vi "ncs_v2.vi"() -> ()   [LabVIEW 2016]
uses:
  <instrlib>/niUSRP/niUSRP Timestamp.ctl
  <vilib>/Analysis/coordinate.llb/Wrap Angle (array).vi
  <instrlib>/niUSRP/niUSRP Configure Time Start Trigger.vi
  <vilib>/Analysis/3filter.llb/Butterworth Filter (DBL).vi
  <instrlib>/niUSRP/niUSRP Fetch Rx Data (2D CDB).vi
  <vilib>/measure/maspectr.llb/FFT Power Spectrum for 1 Chan (CDB).vi
  <instrlib>/niUSRP/niUSRP Write Tx Data (2D CDB).vi
  <vilib>/measure/NI_MABase.lvlib
  <vilib>/measure/NI_MAPro.lvlib
  <vilib>/Analysis/NI_AALBase.lvlib
  <vilib>/Analysis/NI_AALPro.lvlib
  <vilib>/Analysis/NI_AAL_Angle.lvlib
panel:
  in  "File Name":string="Test"
  in  "order1":i32=5
  in  "Order":dbl=20.0 format="%#_13g"
  in  "Path":path=path "D:/Research/SummerFall17Spring18/CnC/NCS/MotionDetectionSleep/MyExperiment/Labview"
  in  "Low-Pass Freq":dbl=200.0 format="%#_13g"
  out "NCS magnitude filtered":dbl[](graph)
  in  "High-Cutoff":dbl=8.0 format="%#_13g"
  in  "Initialize Array-based filter":bool
  in  "Low-Cutoff":dbl=0.5 format="%#_13g"
  in  "Sampling Rate":i32=500
  out "Gain":dbl=-15.0
  out "Bandwidth":dbl=56000000.0
  out "Coerced Carrier Frequency":dbl=2000000000.0 format="%#.17g"
  out "Coerced Tx IQ rate":dbl=1000000.0
  out "Coerced Rx IQ rate":dbl=1000000.0
  out "error IO":errorcluster={"status"=FALSE, "code"=-1074118647, "source"=""}
  in  "Rx Number of Samples":i32=20000
  in  "Tab Control 2":enum32{"NI-294x/295x", "NI-2900/2901"}(tab)=enum."NI-2900/2901"
  in  "channel 0 carrier\n frequency [Hz]":dbl=2000000000.0 format="%#_6p"
  in  "Rx carrier frequency [Hz]":dbl=2000000000.0 format="%#_6p"
  in  "Tx carrier frequency [Hz]":dbl=1000000000.0 format="%#_6p"
  in  "Start Trigger Time":T1={"whole seconds"=1, "fractional seconds"=0.0}
  out "Tx Active Antenna":string="TX1"
  in  "Tab Control":T2(tab)
  out "NCS tag Amp":dbl[](graph)=[0.011967714738528729, 0.012021355192189592, 0.012015275039596582, 0.011969166030167903, 0.011958890166168242, 0.012007893820858737, 0.012022893722444085, 0.011978222225113794, 0.011969989939463181, 0.012003099640895068]
  out "NCS tag Phase":dbl[](graph)=[0.011967714738528729, 0.012021355192189592, 0.012015275039596582, 0.011969166030167903, 0.011958890166168242, 0.012007893820858737, 0.012022893722444085, 0.011978222225113794, 0.011969989939463181, 0.012003099640895068]
  out "IQ":dbl[][](graph)
  out "Tag Amp":dbl[](graph)
  out "Tag Phase":dbl[](graph)
  out "Baseband Power Spectrum":cluster{"f0":dbl, "df":dbl, "magnitude":dbl[]}[](graph)
  in  "Stop":bool
  in  "Channel 0\nTone Amplitude":dbl=0.707 step=0.05 format="%#.6g"
  in  "Channel 0 \nTone Frequency":dbl=5000.0 format="%#_6p"
  out "Tx Waveform Graph":waveform(dbl)[](graph)
  in  "Waveform Size":dbl=2000.0
  in  "Rx Active Antenna":string="RX2"
  in  "Device Name":refnum<k15>="MyB200"
  in  "Tx Gain":dbl=28.0 format="%#_6f"
  in  "Tx IQ Rate":dbl=1000000.0 format="%#_6p"
  in  "Rx Gain":dbl=32.0 format="%#_6f"
  in  "Rx IQ Rate":dbl=1000000.0 format="%#_6p"
  # "Rx Settings"
  # "Tx Settings"
  # "Note that on the NI-2900 and NI-2901, both Rx channels share an LO and both Tx channels share an LO. However, on the NI-294x/295x devices, Rx and Tx of channel 0 share an LO and Rx and Tx of channel 1 share an LO."
  # "This Tx graph should always have end and start tied up since this is being sent in a loop continuously. Otherwise phase jumps will be noticed."
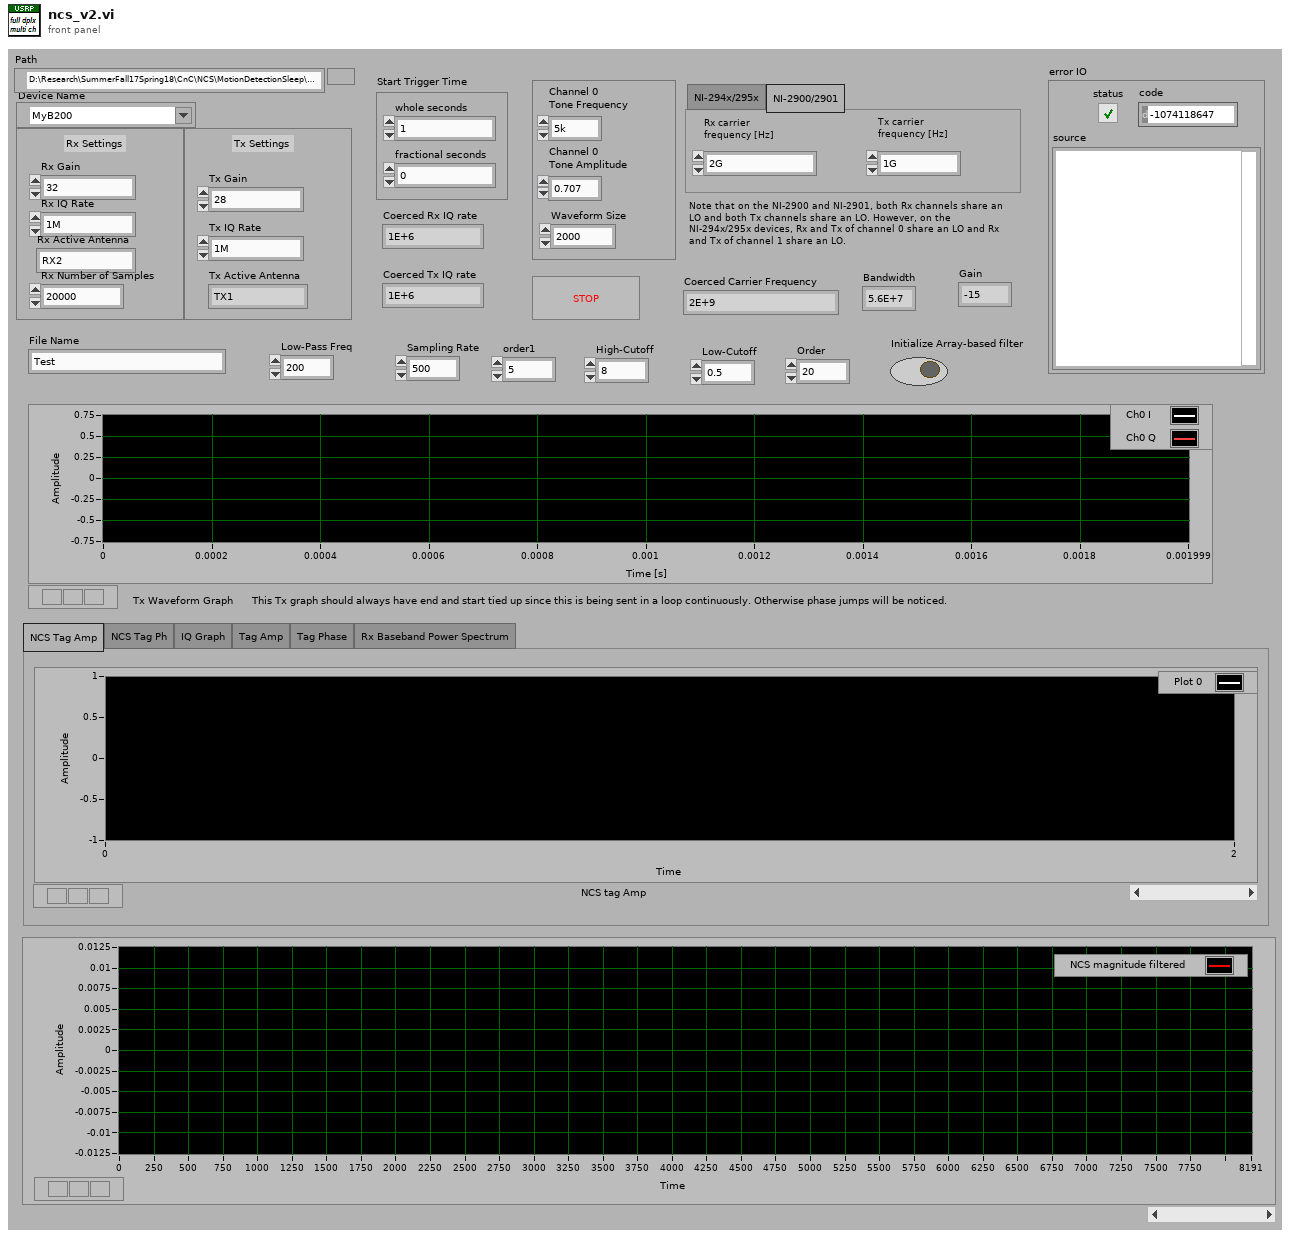
[diagram p1: front panel]
types:
  T1 = typedef "niUSRP Timestamp.ctl" = cluster{"whole seconds":u64, "fractional seconds":dbl}
  T2 = enum32{"NCS Tag Amp", "NCS Tag Ph", "IQ Graph", "Tag Amp", "Tag Phase", "Rx Baseband Power Spectrum"}
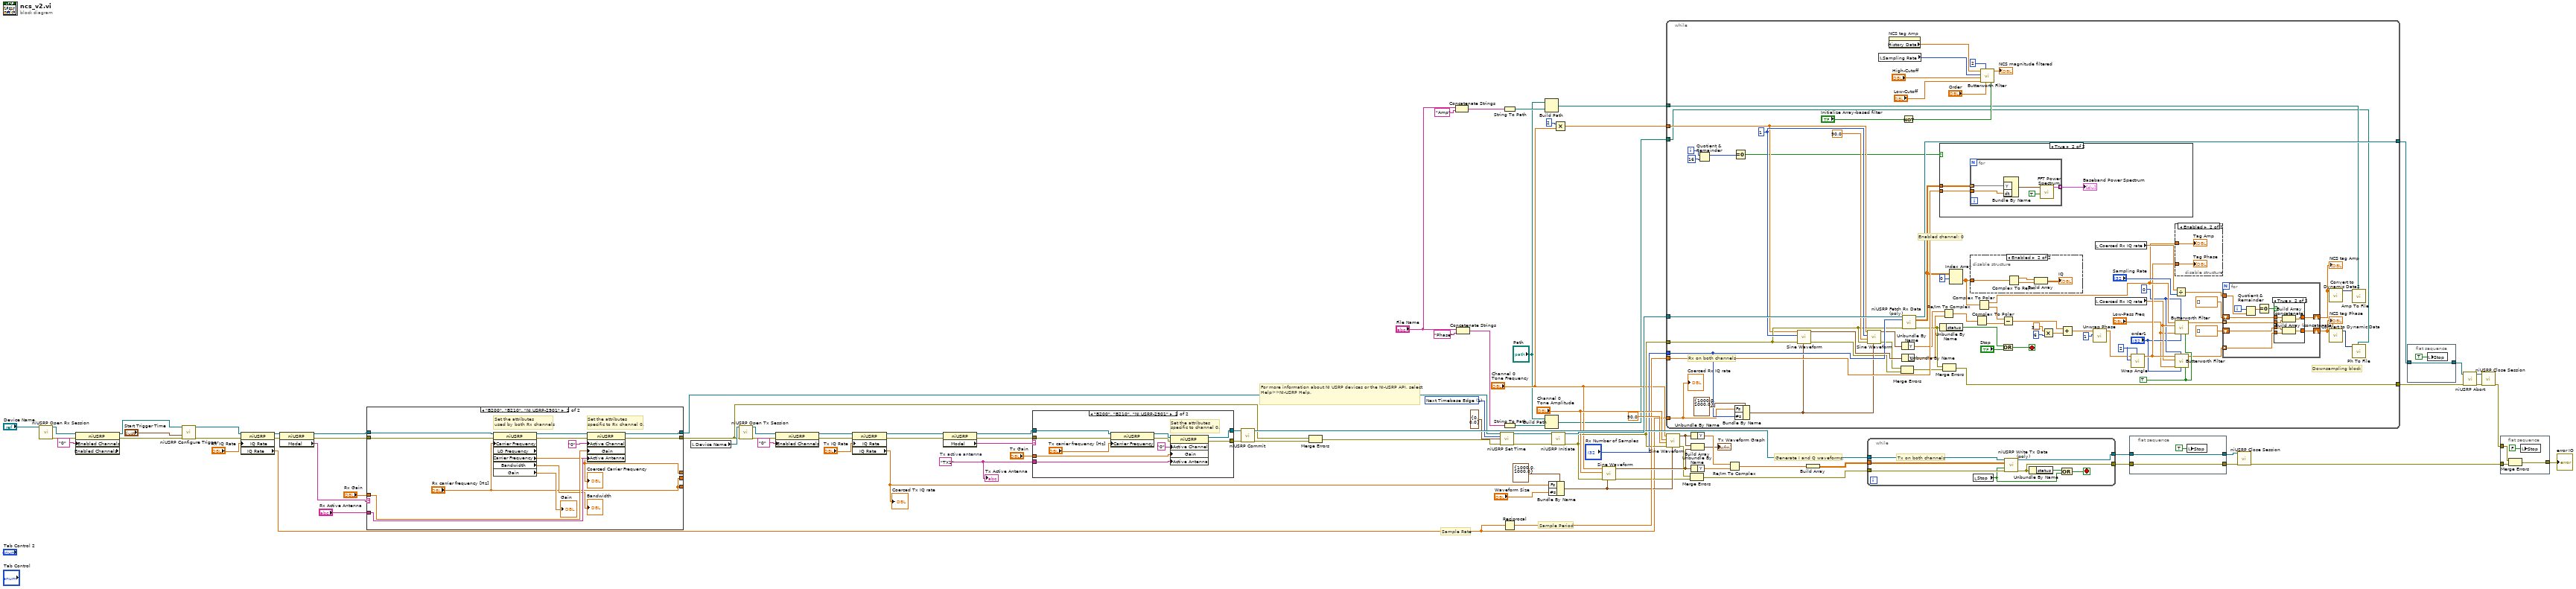
[diagram p0: block diagram]
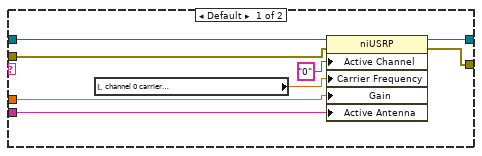
[diagram p2: hidden frame]
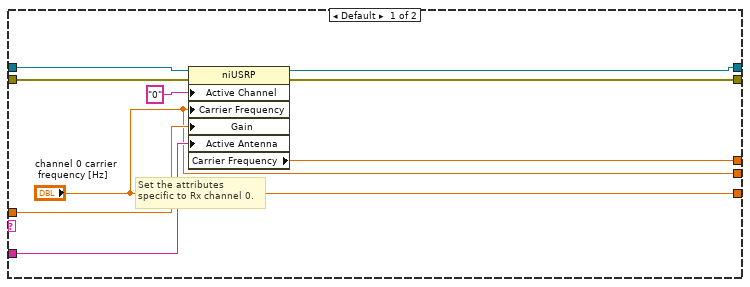
[diagram p3: hidden frame]
diagram:
  w61 = 1 items=["Now", "Next Timebase Edge"] ("apply timestamp")
  w30 = "TX1"  # Tx active antenna
  # "Sample Rate"
  # "Sample Period"
  # "For more information about NI USRP devices or the NI-USRP API, select Help>>NI-USRP Help."
  # "Generate I and Q waveforms."
  n1 = call <instrlib>:"niUSRP Open Rx Session.vi"("device names"="Device Name") -> ("session handle out"=w60:refnum<k15>, "error out"=w59:errorcluster)  [unwired: 13 in]
  n2 = property class="niUSRP" props=["Enabled Channels", "Enabled Channels"](reference=w60, error in=w59, "Enabled Channels"="0" ("Configuration:Enabled Channels")) -> (reference out=w58:refnum<k15>, error out=w57:errorcluster)  [unwired: 1 out]
  n3 = call-poly <instrlib>:"niUSRP Configure Trigger.vi"("session handle"=w58, "start trigger time"="Start Trigger Time", "error in (no error)"=w57) -> ("session handle out"=w54:refnum<k15>, "error out"=w53:errorcluster)  [unwired: 11 in]
  n4 = property class="niUSRP"(reference=w54, error in=w53, "IQ Rate"="Rx IQ Rate") -> (reference out=w50:refnum<k15>, error out=w51:errorcluster, "IQ Rate"=w15:dbl)
  n5 = property class="niUSRP"(reference=w50, error in=w51) -> (reference out=w45:refnum<k15>, error out=w46:errorcluster, "Model"=w47:string)
  n6 = case shown="\"B200\", \"B210\", \"NI USRP-2901\"" w47 {
    tunnel: w46 -> [w96 w106]
    tunnel: w45 -> [w95 w107]
    tunnel: [w92 w103] -> w49
    tunnel: [w91 w102] -> w48
    tunnel: "Rx Gain" -> [w94 w109]
    tunnel: "Rx Active Antenna" -> [w93 w108]
    tunnel: [w89 w98] -> _
    tunnel: ["channel 0 carrier\n frequency [Hz]" "Rx carrier frequency [Hz]"] -> _
    tunnel: ["channel 0 carrier\n frequency [Hz]" "Rx carrier frequency [Hz]"] -> _
    frame Default {
      # "Set the attributes \nspecific to Rx channel 0."
      n7 = property class="niUSRP"(reference=w95, error in=w96, "Active Channel"="0", "Carrier Frequency"="channel 0 carrier\n frequency [Hz]", "Gain"=w94, "Active Antenna"=w93) -> (reference out=w92:refnum<k15>, error out=w91:errorcluster, "Carrier Frequency"=w89:dbl)
    }
    frame "B200", "B210", "NI USRP-2901" {
      # "Set the attributes \nused by both Rx channels"
      # "Set the attributes \nspecific to Rx channel 0."
      n8 = property class="niUSRP" props=["Carrier Frequency", "LO Frequency", "Carrier Frequency", "Bandwidth", "Gain"](reference=w107, error in=w106, "Carrier Frequency"="Rx carrier frequency [Hz]") -> (reference out=w105:refnum<k15>, error out=w104:errorcluster, "Carrier Frequency"=w98:dbl, "Bandwidth"=→"Bandwidth":dbl, "Gain"=→"Gain":dbl)  [unwired: 1 out]
      "Coerced Carrier Frequency" <- w98
      n9 = property class="niUSRP"(reference=w105, error in=w104, "Active Channel"="0", "Gain"=w109, "Active Antenna"=w108) -> (reference out=w103:refnum<k15>, error out=w102:errorcluster)
    }
  }
  n10 = local read "Device Name"() -> (w82:refnum<k15>)
  n11 = call <instrlib>:"niUSRP Open Tx Session.vi"("device names"=w82, "error in (no error)"=w48) -> ("session handle out"=w56:refnum<k15>, "error out"=w55:errorcluster)  [unwired: 12 in]
  n12 = property class="niUSRP"(reference=w56, error in=w55, "Enabled Channels"="0" ("Configuration:Enabled Channels")) -> (reference out=w42:refnum<k15>, error out=w41:errorcluster)
  n13 = property class="niUSRP"(reference=w42, error in=w41, "IQ Rate"="Tx IQ Rate") -> (reference out=w36:refnum<k15>, error out=w37:errorcluster, "IQ Rate"=w34:dbl)
  "Coerced Tx IQ rate" <- w34
  n14 = property class="niUSRP"(reference=w36, error in=w37) -> (reference out=w38:refnum<k15>, error out=w39:errorcluster, "Model"=w35:string)
  n15 = case shown="\"B200\", \"B210\", \"NI USRP-2901\"" w35 {
    tunnel: "Tx Gain" -> [w118 w128]
    tunnel: w30 -> [w116 w126]
    tunnel: [w112 w120] -> w32
    tunnel: [w111 w119] -> w33
    tunnel: w39 -> [w115 w122]
    tunnel: w38 -> [w114 w125]
    frame Default {
      n16 = local read "channel 0 carrier\n frequency [Hz]"() -> (w113:dbl)
      n17 = property class="niUSRP"(reference=w114, error in=w115, "Active Channel"="0", "Carrier Frequency"=w113, "Gain"=w118, "Active Antenna"=w116) -> (reference out=w112:refnum<k15>, error out=w111:errorcluster)
    }
    frame "B200", "B210", "NI USRP-2901" {
      # "Set the attributes \nspecific to channel 0."
      n18 = property class="niUSRP"(reference=w125, error in=w122, "Carrier Frequency"="Tx carrier frequency [Hz]") -> (reference out=w124:refnum<k15>, error out=w123:errorcluster)
      n19 = property class="niUSRP"(reference=w124, error in=w123, "Active Channel"="0", "Gain"=w128, "Active Antenna"=w126) -> (reference out=w120:refnum<k15>, error out=w119:errorcluster)
    }
  }
  n20 = call <instrlib>:"niUSRP Commit.vi"("session handle"=w32, "error in (no error)"=w33) -> ("session handle out"=w84:refnum<k15>, "error out"=w85:errorcluster)  [unwired: 12 in]
  n21 = Merge Errors(w48, w85) -> (w63:errorcluster)
  n22 = Concatenate Strings("File Name", "Amp") -> (w8:string)
  n23 = Concatenate Strings("File Name", "Phase") -> (w4:string)
  n24 = call <instrlib>:"niUSRP Set Time.vi"("session handle"=w49, "apply timestamp"=w61, "timestamp"=T1 {"whole seconds"=0, "fractional seconds"=0.0}, "error in (no error)"=w63) -> ("session handle out"=w65:refnum<k15>, "error out"=w64:errorcluster)  [unwired: 10 in]
  n25 = String To Path(string=w8) -> (path=w7:path)
  n26 = String To Path(string=w4) -> (path=w3:path)
  n27 = Reciprocal(x=w15) -> (1/x=w68:dbl)
  n28 = Build Path(base path="Path", name or relative path=w7) -> (appended path=w10:path)
  n29 = Build Path(base path="Path", name or relative path=w3) -> (appended path=w1:path)
  n30 = Bundle By Name(cluster=cluster{"Fs":dbl, "#s":dbl} {"Fs"=1000.0, "#s"=1000.0} ("sampling info"), "Fs"=w34, "#s"="Waveform Size") -> (w67:cluster{"Fs":dbl, "#s":dbl})
  n31 = call <instrlib>:"niUSRP Initiate.vi"("session handle"=w65, "error in (no error)"=w64) -> ("session handle out"=w88:refnum<k15>, "error out"=w29:errorcluster)  [unwired: 12 in]
  n32 = Multiply(x=2, y="Channel 0 \nTone Frequency") -> (x*y=w12:dbl)
  n33 = call <vilib>:"Sine Waveform.vi"("sampling info"=w67, "error in (no error)"=w29, "amplitude"="Channel 0\nTone Amplitude", "frequency"="Channel 0 \nTone Frequency") -> ("error out"=w28:errorcluster, "signal out"=w77:waveform(dbl))  [unwired: 6 in]
  n34 = while {
    tunnel: w88 -> [w198]
    tunnel: w29 -> [w185]
    tunnel: [w197] -> w22
    tunnel: w68 -> [w192]
    tunnel: "Rx Number of Samples" -> [w189]
    tunnel: w15 -> [w179]
    tunnel: w12 -> [w180]
    tunnel: [w160] -> w11
    tunnel: w10 -> [w157]
    tunnel: w1 -> [w132]
    i -> [w158]
    stop <- w161 stop-if-true
    w144 = 2 ("y")
    w137 = TRUE
    w139 = 0
    w187 = 1
    # "Downsampling block"
    # "Enabled channel: 0"
    # "Rx on both channels"
    n35 = Quotient & Remainder(x=w158, y=16) -> (x-y*floor(x/y)=w196:i32)  [unwired: 1 out]
    n36 = Equal To 0?(x=w196) -> (x = 0?=w159:bool)
    n37 = Bundle By Name(cluster=cluster{"Fs":dbl, "#s":dbl} {"Fs"=1000.0, "#s"=1000.0} ("sampling info"), "Fs"=w179, "#s"=w189) -> (w186:cluster{"Fs":dbl, "#s":dbl})
    n38 = call <vilib>:"Sine Waveform.vi"("sampling info"=w186, "error in (no error)"=w185, "amplitude"=w187, "frequency"=w180) -> ("error out"=w184:errorcluster, "signal out"=w190:waveform(dbl))  [unwired: 6 in]
    n39 = call <vilib>:"Sine Waveform.vi"("sampling info"=w186, "error in (no error)"=w185, "phase"=90.0, "amplitude"=w187, "frequency"=w180) -> ("error out"=w183:errorcluster, "signal out"=w181:waveform(dbl))  [unwired: 5 in]
    n40 = local read "Sampling Rate"() -> (w163:i32)
    n41 = property on="NCS tag Amp" class="WaveformChart (strict)"() -> ("History Data"=w167:dbl[])  [unwired: 2 in, 2 out]
    n42 = Merge Errors(w183, w184) -> (w182:errorcluster)
    n43 = Unbundle By Name(w181) -> ("Y"=w154:dbl[])
    n44 = Unbundle By Name(w190) -> ("Y"=w153:dbl[])
    n45 = Not(x="Initialize Array-based filter") -> (.not. x?=w168:bool)
    n46 = call-poly <instrlib>:"niUSRP Fetch Rx Data (poly).vi"("session handle"=w198, "number of samples"=w189, "error in (no error)"=w185) -> ("session handle out"=w197:refnum<k15>, "data"=w177:cdb[][], "error out"=w169:errorcluster)  [unwired: 9 in, 1 out]
    n47 = case shown="True" w159 {
      tunnel: w177 -> [_ w225]
      tunnel: w192 -> [_ w224]
      frame False {
      }
      frame True {
        n48 = for {
          tunnel: w225 -> [w228] mode=indexing
          tunnel: w224 -> [w227]
          tunnel: [w226] -> w223 mode=indexing
          n49 = Bundle By Name("Y"=w228, "dt"=w227) -> (w229:waveform(cdb))  [unwired: 1 in]
          n50 = call-poly <vilib>:"FFT Power Spectrum.vi"("dB On (F)"=TRUE, "time signal"=w229) -> ("power spectrum"=w226:cluster{"f0":dbl, "df":dbl, "magnitude":dbl[]})  [unwired: 6 in, 3 out]
        }
        "Baseband Power Spectrum" <- w223
      }
    }
    n51 = Unbundle By Name(w169) -> ("status"=w194:bool)
    n52 = Re/Im To Complex(1:w153, 2:w154) -> (0:w147:cdb[])
    n53 = Merge Errors(w169, w182) -> (w160:errorcluster)
    n54 = Index Array(array=w177, index (row)=0 ("y")) -> (element=w176:cdb[])  [unwired: 1 in]
    n55 = disable-structure shown="Enabled" {
      disable-tunnel: w176 -> [_ w201]
      frame Disabled {
      }
      frame Enabled {
        n56 = Complex To Re/Im(x + iy=w201) -> (x=w204:dbl[], y=w203:dbl[])
        n57 = Build Array(w204, w203) -> (→"IQ":dbl[][])
      }
    }
    n58 = Complex To Polar(r * e^(i*theta)=w147) -> (theta=w148:dbl[])  [unwired: 1 out]
    n59 = Complex To Polar(r * e^(i*theta)=w176) -> (r=w156:dbl[], theta=w142:dbl[])
    n60 = call-poly <vilib>:"Butterworth Filter.vi"("init/cont (init:F)"=w168, "order"="Order", "filter type"=2, "low cutoff freq: fl"="Low-Cutoff", "high cutoff freq: fh"="High-Cutoff", "sampling freq: fs"=w163, "X"=w167) -> ("Filtered X"=→"NCS magnitude filtered":dbl[])  [unwired: 1 in, 1 out]
    n61 = Subtract(x=w142, y=w148) -> (x-y=w146:dbl[])
    n62 = Or(x=w194, y="Stop") -> (x .or. y?=w161:bool)
    n63 = Multiply(x=3.141592653589793, y=6) -> (x*y=w149:dbl)
    n64 = Add(x=w146, y=w149) -> (x+y=w145:dbl[])
    n65 = call <vilib>:"Unwrap Phase.vi"("phase unit"=1 ("y"), "Phase"=w145) -> ("Unwrapped Phase"=w143:dbl[])  [unwired: 8 in, 1 out]
    n66 = local read "Coerced Rx IQ rate"() -> (w166:dbl)
    n67 = local read "Coerced Rx IQ rate"() -> (w140:dbl)
    n68 = call-poly <vilib>:"Wrap Angle.vi"("angle units"=w144, "angle range"=w144, "Angle In"=w143) -> ("Angle Out"=w141:dbl[])  [unwired: 7 in, 1 out]
    n69 = Divide(x=w166, y="Sampling Rate") -> (x/y=w164:dbl)
    n70 = disable-structure shown="Enabled" {
      disable-tunnel: w156 -> [_ w200]
      disable-tunnel: w141 -> [_ w199]
      frame Disabled {
      }
      frame Enabled {
        "Tag Amp" <- w200
        "Tag Phase" <- w199
      }
    }
    n71 = call-poly <vilib>:"Butterworth Filter.vi"("init/cont (init:F)"=w137, "order"="order1", "filter type"=w139, "low cutoff freq: fl"="Low-Pass Freq", "sampling freq: fs"=w140, "X"=w156) -> ("Filtered X"=w155:dbl[])  [unwired: 2 in, 1 out]
    n72 = call-poly <vilib>:"Butterworth Filter.vi"("init/cont (init:F)"=w137, "order"="order1", "filter type"=w139, "low cutoff freq: fl"="Low-Pass Freq", "sampling freq: fs"=w140, "X"=w141) -> ("Filtered X"=w135:dbl[])  [unwired: 2 in, 1 out]
    n73 = for {
      tunnel: w155 -> [w214] mode=indexing
      shift-right: [w212] -> w130
      shift-left: dbl[] [] -> [w213]
      tunnel: w164 -> [w208]
      shift-right: [w206] -> w133
      shift-left: dbl[] [] -> [w207]
      tunnel: w135 -> [w205] mode=indexing
      i -> [w211]
      n74 = Quotient & Remainder(x=w211, y=w208) -> (x-y*floor(x/y)=w209:dbl)  [unwired: 1 out]
      n75 = Equal To 0?(x=w209) -> (x = 0?=w210:bool)
      n76 = case shown="True" w210 {
        tunnel: w214 -> [_ w222]
        tunnel: w213 -> [w216 w221]
        tunnel: [w216 w220] -> w212
        tunnel: w207 -> [w215 w219]
        tunnel: [w215 w218] -> w206
        tunnel: w205 -> [_ w217]
        frame False {
        }
        frame True {
          n77 = Build Array (concatenate)(w221, w222) -> (w220:dbl[])
          n78 = Build Array (concatenate)(w219, w217) -> (w218:dbl[])
        }
      }
    }
    "NCS tag Amp" <- w130
    "NCS tag Phase" <- w133
    n79 = call "Convert to Dynamic Data2"("Array"=w130) -> ("Dynamic Data Type"=w129:dynamicdata)  [unwired: 3 in]
    n80 = call "Convert to Dynamic Data"("Array"=w133) -> ("Dynamic Data Type"=w134:dynamicdata)  [unwired: 3 in]
    n81 = call "Amp To File"("Signals"=w129, "Filename"=w157) -> ()  [unwired: 15 in, 3 out]
    n82 = call "Ph To File"("Signals"=w134, "Filename"=w132) -> ()  [unwired: 15 in, 3 out]
    "Coerced Rx IQ rate" <- w179
  }
  n83 = call <vilib>:"Sine Waveform.vi"("sampling info"=w67, "error in (no error)"=w29, "phase"=90.0, "amplitude"="Channel 0\nTone Amplitude", "frequency"="Channel 0 \nTone Frequency") -> ("error out"=w27:errorcluster, "signal out"=w76:waveform(dbl))  [unwired: 5 in]
  n84 = Merge Errors(w27, w28) -> (w26:errorcluster)
  n85 = Unbundle By Name(w76) -> ("Y"=w75:dbl[])
  n86 = Build Array(w76, w77) -> (→"Tx Waveform Graph":waveform(dbl)[])
  n87 = Unbundle By Name(w77) -> ("Y"=w74:dbl[])
  n88 = Re/Im To Complex(1:w74, 2:w75) -> (0:w70:cdb[])
  n89 = Build Array(w70) -> (w69:cdb[][])
  n90 = while {
    tunnel: w84 -> [w238]
    tunnel: w26 -> [w237]
    tunnel: [w235] -> w25
    tunnel: [w233] -> w20
    tunnel: w69 -> [w231]
    stop <- w234 stop-if-true
    # "Tx on both channels"
    n91 = local read "Stop"() -> (w232:bool)
    n92 = call-poly <instrlib>:"niUSRP Write Tx Data (poly).vi"("session handle"=w238, "data"=w231, "end of data?"=w232, "error in (no error)"=w237) -> ("session handle out"=w233:refnum<k15>, "error out"=w235:errorcluster)  [unwired: 10 in]
    n93 = Unbundle By Name(w235) -> ("status"=w236:bool)
    n94 = Compound Arithmetic op=OR(w236, w232) -> (w234:bool)
  }
  n95 = flat-sequence {
    tunnel: [w240] -> w24
    tunnel: w25 -> [w240]
    tunnel: [w239] -> w21
    tunnel: w20 -> [w239]
    frame #0 {
      n96 = local write "Stop"(TRUE ("STOP")) -> ()
    }
  }
  n97 = call <instrlib>:"niUSRP Close Session.vi"("session handle"=w21, "error in (no error)"=w24) -> ("error out"=w19:errorcluster)  [unwired: 13 in]
  n98 = flat-sequence {
    tunnel: [w242] -> w23
    tunnel: w22 -> [w242]
    frame #0 {
      n99 = local write "Stop"(TRUE ("STOP")) -> ()
    }
  }
  n100 = call <instrlib>:"niUSRP Abort.vi"("session handle"=w23, "error in (no error)"=w11) -> ("session handle out"=w81:refnum<k15>, "error out"=w80:errorcluster)  [unwired: 12 in]
  n101 = call <instrlib>:"niUSRP Close Session.vi"("session handle"=w81, "error in (no error)"=w80) -> ("error out"=w16:errorcluster)  [unwired: 13 in]
  n102 = flat-sequence {
    tunnel: w19 -> [w246]
    tunnel: [w245] -> w17
    tunnel: w16 -> [w244]
    frame #0 {
      n103 = Merge Errors(w244, w246) -> (w245:errorcluster)
      n104 = local write "Stop"(FALSE ("STOP")) -> ()
    }
  }
  "Tx Active Antenna" <- w30
  "error IO" <- w17
